vi "IMAQdx Write Register2.vi"(8 "error in":errorcluster, 9 "Value":u32 format="%.0x", 10 "Offset":u64=4042262528 format="%.0x", 11 "Session In":T1) -> (0 "error out":errorcluster, 3 "Session Out":T1)   [LabVIEW 2020, in "NI_Vision_Acquisition_Software.lvlib"]
doc: "Accesses registers on the camera and writes a 32-bit value to the camera. Data is byte-swapped for big endian alignment before transfer."
uses:
  NI_Vision_Acquisition_Software.lvlib
  IMAQdx.ctl
  niimaqdx.dll
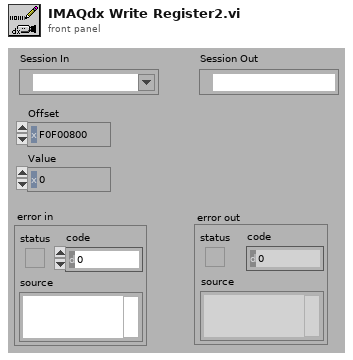
[diagram p1: front panel]
types:
  T1 = typedef "IMAQdx.ctl" = refnum<k21>
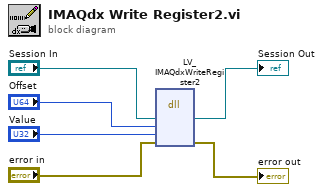
[diagram p0: block diagram]
diagram:
  n1 = dll-call lib="niimaqdx.dll" fn="LV_IMAQdxWriteRegister2"("refNum"="Session In", "offset"="Offset", "value"="Value", "err"="error in") -> ("refNum"=→"Session Out":T1, "err"=→"error out":errorcluster)  [unwired: 6 in, 2 out]
